vi "PV Date of listed errors.vi"(0 "VISA session":refnum<visa-resource-name>, 5 "Adress of unit":u16=1 min=1 max=999 step=1, 7 "Position :":u16=1 min=1 max=10 step=1, 11 "error in (no error)":errorcluster) -> (4 "dup VISA session":refnum<visa-resource-name>, 6 "response (data)":string, 15 "error out":errorcluster)   [LabVIEW 2016, in "Pfeiffer Vacuum.lvlib"]
doc: "Read Time / Date of listed error storage at Position 1 - 10 .\nParameter: 370 - 379\n\nValid Range 1 to 10\nDefault Value: 1"
uses:
  Pfeiffer Vacuum.lvlib
panel:
  # "Read Time/Date of listed \nerror storage at"
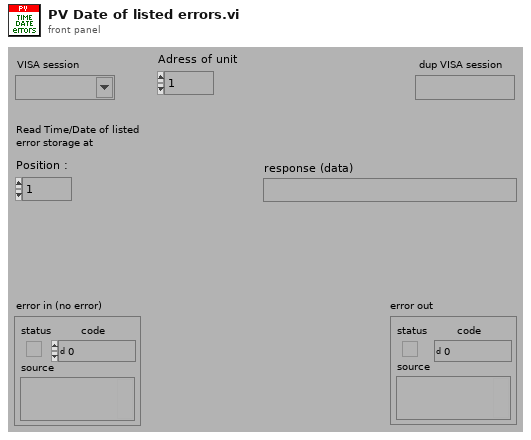
[diagram p1: front panel]
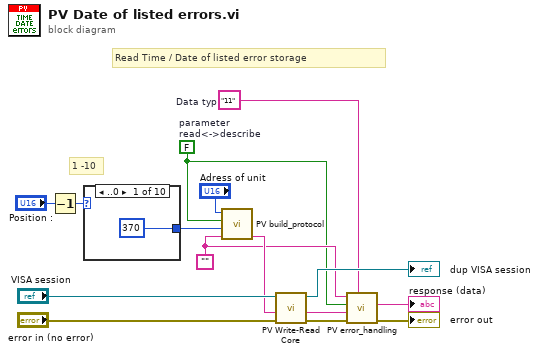
[diagram p0: block diagram]
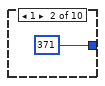
[diagram p2: hidden frame]
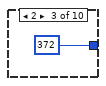
[diagram p3: hidden frame]
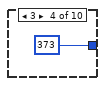
[diagram p4: hidden frame]
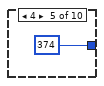
[diagram p5: hidden frame]
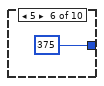
[diagram p6: hidden frame]
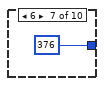
[diagram p7: hidden frame]
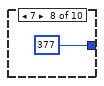
[diagram p8: hidden frame]
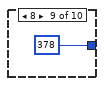
[diagram p9: hidden frame]
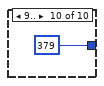
[diagram p10: hidden frame]
diagram:
  w3 = "11"  # Data typ
  w2 = ""
  w1 = FALSE  # parameter read<->describe
  # "1 -10"
  # "Read Time / Date of listed error storage"
  n1 = Decrement(x="Position :") -> (x-1=w12:u16)
  n2 = case shown="..0" w12 {
    tunnel: [u16 370 ("Parameter-number") u16 371 ("Parameter-number") u16 372 ("Parameter-number") u16 373 ("Parameter-number") u16 374 ("Parameter-number") u16 375 ("Parameter-number") u16 376 ("Parameter-number") u16 377 ("Parameter-number") u16 378 ("Parameter-number") u16 379 ("Parameter-number")] -> w14
    frame ..0 {
    }
    frame 1 {
    }
    frame 2 {
    }
    frame 3 {
    }
    frame 4 {
    }
    frame 5 {
    }
    frame 6 {
    }
    frame 7 {
    }
    frame 8 {
    }
    frame 9.. {
    }
  }
  n3 = call "PV build_protocol.vi"("Data"=w2, "Parameter-number"=w14, "parameter\nread<->describe"=w1, "Adress"="Adress of unit") -> ("output"=w9:string)  [unwired: 3 in]
  n4 = call "PV Write-Read Core.vi"("error in"="error in (no error)", "Write data in"=w9, "VISA session"="VISA session") -> ("error out"=w6:errorcluster, "response (data) out"=w7:string, "dup VISA session"=→"dup VISA session":refnum<visa-resource-name>)  [unwired: 2 in]
  n5 = call "PV error_handling.vi"("Data Typ in"=w3, "error in"=w6, "response (data) in"=w7, "Parameter\nread only<->describe"=w1, "data in"=w2) -> ("error out"=→"error out":errorcluster, "Data out"=→"response (data)":string)  [unwired: 4 in, 1 out]
